vi "Write ROI Ext.vi"(8 "error in (no error)":errorcluster, 10 "ROI Descriptor":T1 {"Contours"."Type" items=["No Selection", "Point", "Line", "Rectangle", "Oval", "Polygon", "Freehand Region", "Annulus", "Unused2", "Unused3", "Broken Line", "Freehand Line", "Rotated Rectangle"]}, 11 "IMAQ Display in":refnum<class "HIJ Vision Display.lvclass">) -> (0 "error out":errorcluster, 3 "IMAQ Display out":refnum<class "HIJ Vision Display.lvclass">)   [LabVIEW 2014, in "HIJ Vision Display.lvlib" / "HIJ Vision Display.lvclass"]
uses:
  HIJ Vision Display.lvclass
  Analyze Parameter/Analyze Parameter ROI/Analyze Parameter ROI.lvclass
  HIJ Vision Display.lvclass/HIJ Vision Display.ctl
  Analyze Parameter/Analyze Parameter ROI/Analyze Parameter ROI.lvclass/Analyze Parameter ROI.ctl
  Analyze Actor/Analyze Actor Messages/Set Analyze Parameter Msg/Set Analyze Parameter Msg.lvclass/Set Analyze Parameter Msg.ctl
  <vilib>/ActorFramework/Message Enqueuer/Message Enqueuer.lvclass/Message Enqueuer.ctl
  Analyze Parameter/Analyze Parameter ROI/Write ROI Descriptor.vi
  <vilib>/ActorFramework/Message Enqueuer/Enqueue.vi
  <vilib>/ActorFramework/Message Priority Queue/Priority Enqueue.vi
  Analyze Actor/Analyze Actor Messages/Set Analyze Parameter Msg/Set Analyze Parameter Msg.lvclass
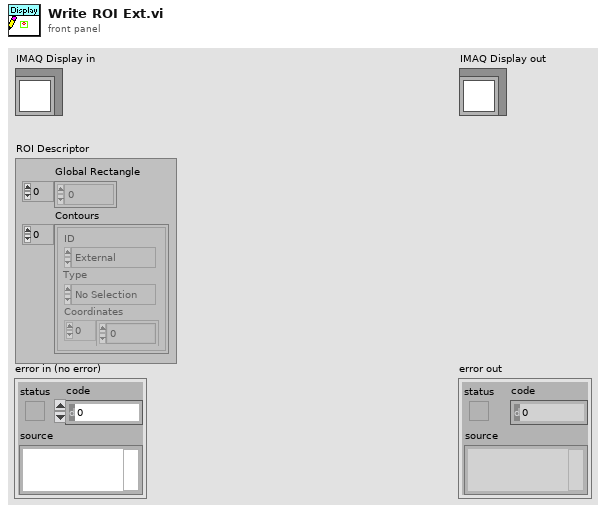
[diagram p1: front panel]
types:
  T1 = typedef "ROI Descriptor" = cluster{"Global Rectangle":i32[], "Contours":cluster{"ID":enum32{"External", "Internal"}, "Type":u32, "Coordinates":i32[]}[]}
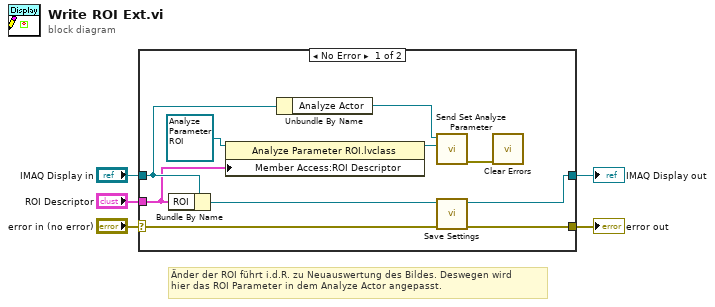
[diagram p0: block diagram]
diagram:
  # "Änder der ROI führt i.d.R. zu Neuauswertung des Bildes. Deswegen wird\nhier das ROI Parameter in dem Analyze Actor angepasst."
  n1 = case shown="No Error" "error in (no error)" {
    selector: "error in (no error)" -> [w13 w16]
    tunnel: [w12 w16] -> w4
    tunnel: [w14 w17] -> w2
    tunnel: "IMAQ Display in" -> [w11 w17]
    tunnel: "ROI Descriptor" -> [w9 _]
    frame No Error {
      n2 = Bundle By Name(cluster=w11, "ROI"=w9) -> (w15:refnum<class "HIJ Vision Display.lvclass">)
      n3 = property class="Analyze Parameter ROI.lvclass"(reference=refnum<class "Analyze Parameter ROI.lvclass"> refnum ("Analyze Parameter ROI.lvclass"), "Member Access:ROI Descriptor"=w9) -> (reference out=w7:refnum<class "Analyze Parameter ROI.lvclass">)  [unwired: 1 in, 1 out]
      n4 = Unbundle By Name(w11) -> ("Analyze Actor"=w8:refnum<class "Message Enqueuer.lvclass">)
      n5 = call "Send Set Analyze Parameter.vi"("Analyze Parameter"=w7, "Message Enqueuer"=w8) -> ("error out"=w6:errorcluster)  [unwired: 8 in, 1 out]
      n6 = call-dynamic "Save Settings.vi"("error in (no error)"=w13, "IMAQ Display in"=w15) -> ("error out"=w12:errorcluster, "IMAQ Display out"=w14:refnum<class "HIJ Vision Display.lvclass">)  [unwired: 8 in]
      n7 = call <vilib>:"Clear Errors.vi"("error in (no error)"=w6) -> ()  [unwired: 5 in, 2 out]
    }
    frame Error {
    }
  }
  "error out" <- w4
  "IMAQ Display out" <- w2
